vi "test8-AsteriskWildcardStatusRegistration.vi"(8 "error in (no error)":errorcluster, 11 "TestCase in":refnum<class "testcase-CSMBroadcast.lvclass">) -> (0 "error out":errorcluster, 3 "TestCase out":refnum<class "testcase-CSMBroadcast.lvclass">)   [LabVIEW 2017, in "testcase-CSMBroadcast.lvclass"]
uses:
  testcase-CSMBroadcast.lvclass
  0c20cacf-7d77-4f8e-aec5-f22e7d09936d.vi
  26de337d-8090-412f-9da5-e117a55d4726.vi
  de10340a-d592-45ad-b055-7fa7b377c551.vi
  e3eae2f8-d8ce-4adb-8167-9a417250fce1.vi
  a4d00e00-a9ed-4631-bf53-269bf71f16fc.vi
  src/user.lib/_NEVSTOP/Communicable State Machine(CSM)/AdvanceAPI/CSM - Revert Arguments-Safe String.vi
  src/user.lib/_NEVSTOP/Communicable State Machine(CSM)/AdvanceAPI/CSM - Make String Arguments Safe.vi
  src/user.lib/_NEVSTOP/Communicable State Machine(CSM)/AdvanceAPI/CSM - Break Down Multiple States String.vi
  src/user.lib/_NEVSTOP/Communicable State Machine(CSM)/AdvanceAPI/CSM - Compact Multiple States.vi
  src/user.lib/_NEVSTOP/Communicable State Machine(CSM)/AdvanceAPI/CSM - Keywords.vi
  src/user.lib/_NEVSTOP/Communicable State Machine(CSM)/_Shared/Trim Single-line Text.vi
  src/user.lib/_NEVSTOP/Communicable State Machine(CSM)/AdvanceAPI/CSM - Set Module Attribute.vi
  src/user.lib/_NEVSTOP/Communicable State Machine(CSM)/AdvanceAPI/CSM - Get Module Attribute.vi
  <vilib>/addons/_JKI Toolkits/VI Tester/TestCase.llb/TestCase.lvclass
  src/user.lib/_NEVSTOP/Communicable State Machine(CSM)/Communicable State Machine.lvlib
  CSM/CSM-Testcase.lvlib
  C:/Program Files (x86)/National Instruments/LabVIEW 2017/vi.lib/addons/_JKI Toolkits/VI Tester/TestCase.llb/TestCase.lvclass
panel:
  out "Execution Times":i32
  out "State History":string
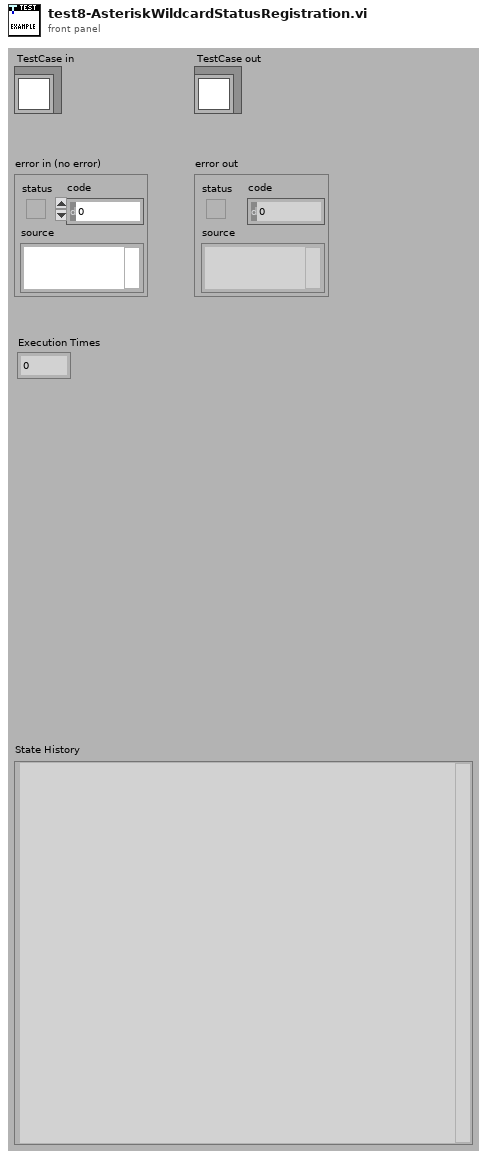
[diagram p1: front panel]
types:
  T1 = enum32{"Invalid", "Standard", "Closed", "Hidden", "Minimized", "Maximized"}
  T2 = enum32{"invalid app kind", "Development System", "Run Time System", "Student Edition", "Embedded LabVIEW", "Evaluation", "Custom"}
  T3 = typedef "Communicable State Machine.lvlib/_CSM_Response Source Message.ctl" = cluster{"‘State":string, "’Arguments":string, "’Error":errorcluster}
  T4 = cluster{"Current VI Reference":refnum<vi>, "Close Panel on Exit?":bool}
  T5 = cluster{"Core":cluster{"Current VI Reference":refnum<vi>, "Close Panel on Exit?":bool}, "Your Boolean data":bool, "Your string data":string, "TestData":i32}
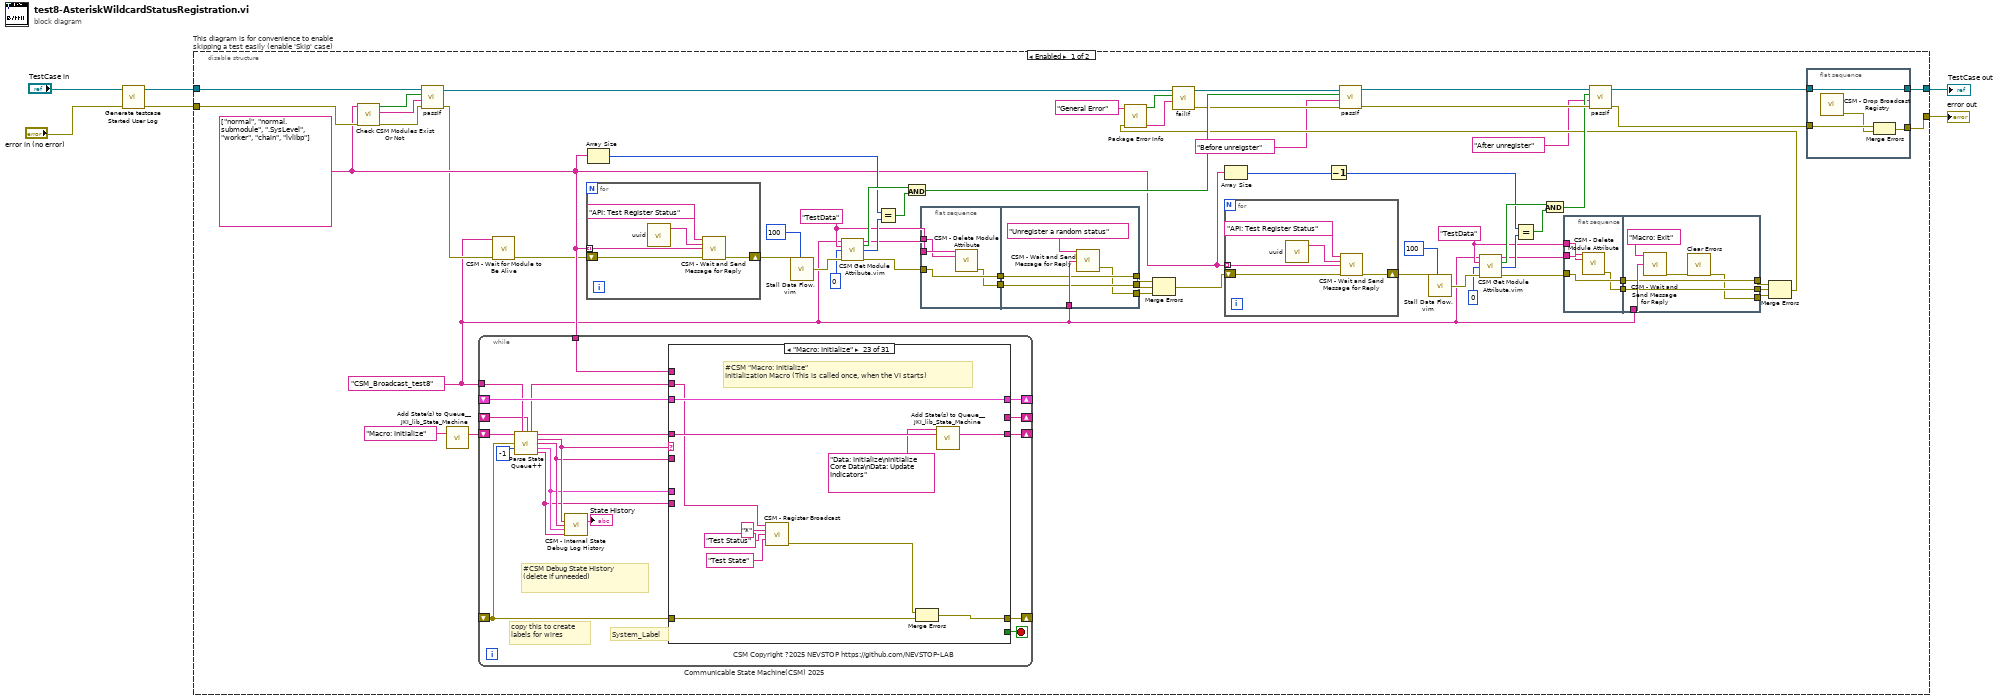
[diagram p0: block diagram]
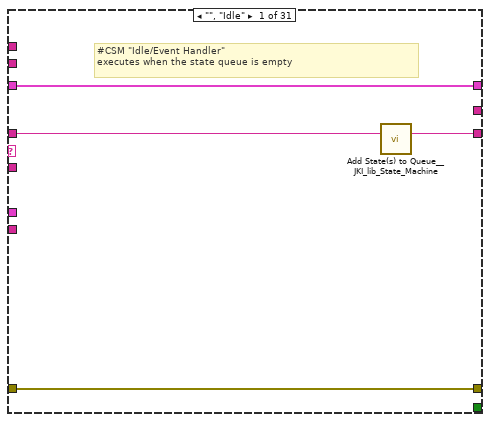
[diagram p2: hidden frame]
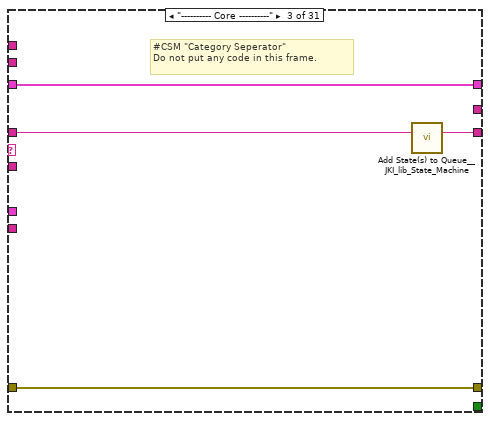
[diagram p4: hidden frame]
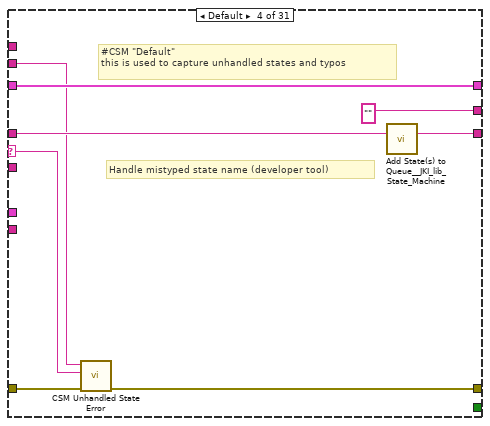
[diagram p5: hidden frame]
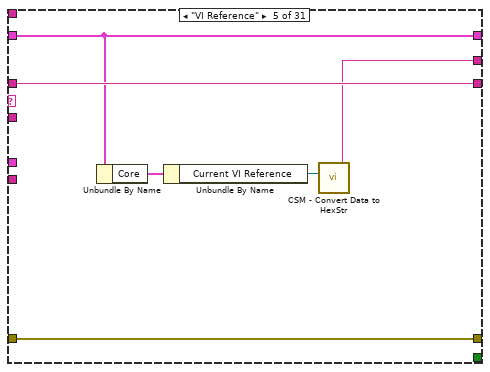
[diagram p6: hidden frame]
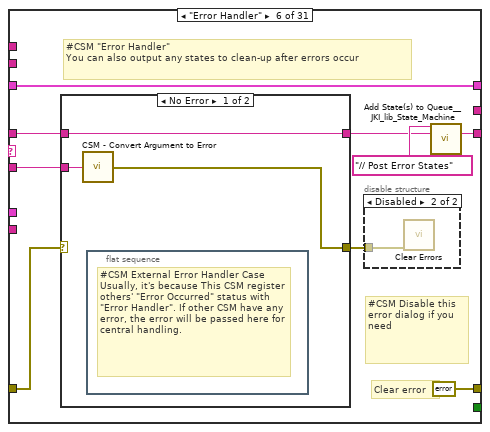
[diagram p7: hidden frame]
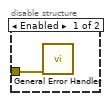
[diagram p8: hidden frame]
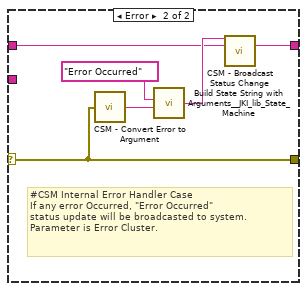
[diagram p9: hidden frame]
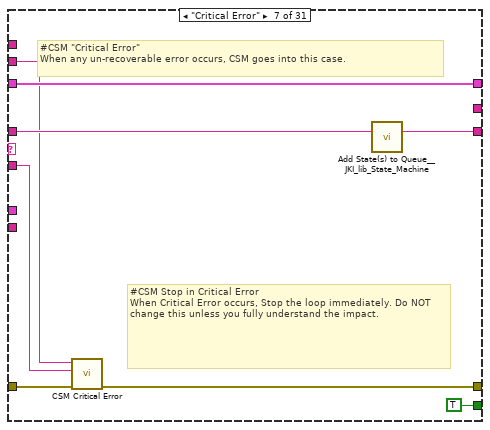
[diagram p10: hidden frame]
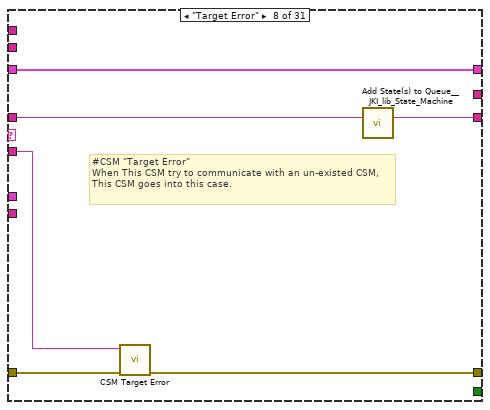
[diagram p11: hidden frame]
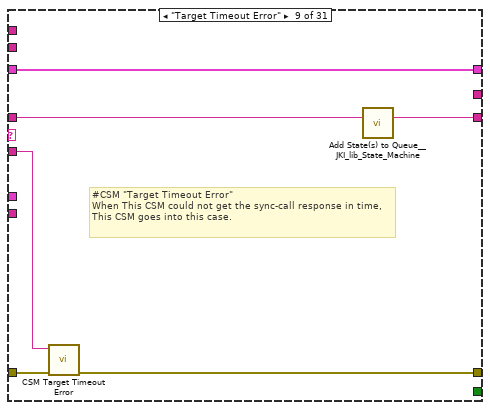
[diagram p12: hidden frame]
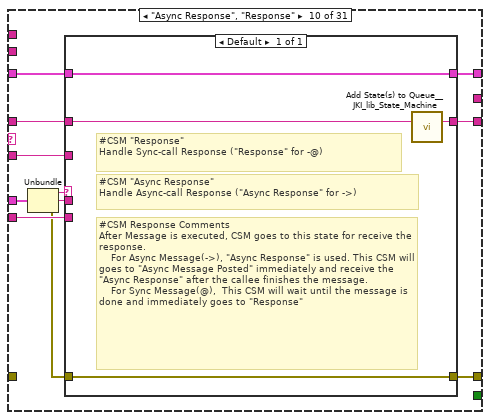
[diagram p13: hidden frame]
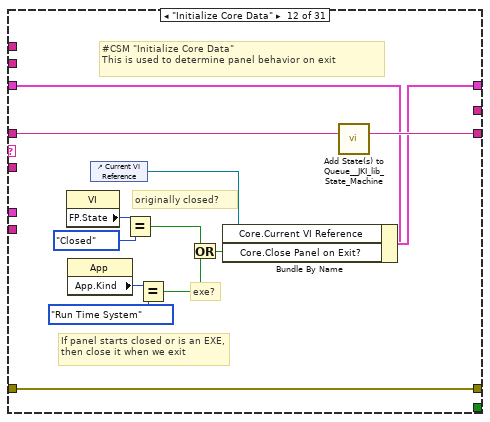
[diagram p15: hidden frame]
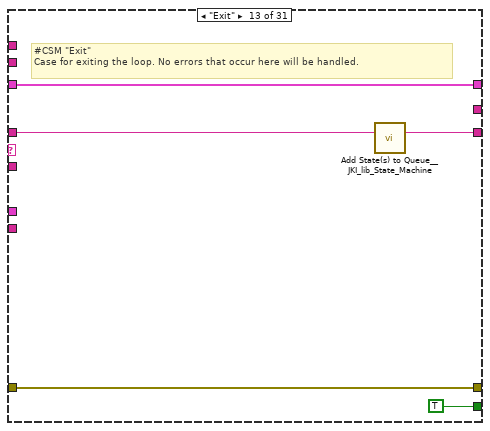
[diagram p16: hidden frame]
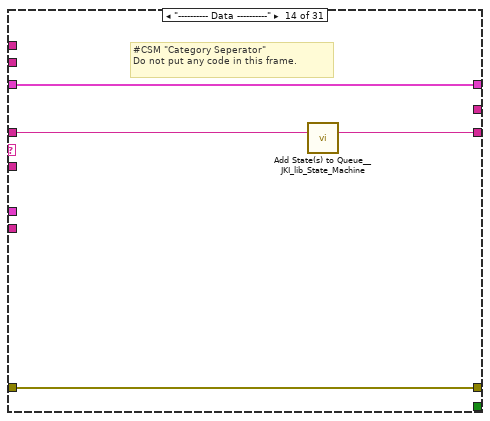
[diagram p17: hidden frame]
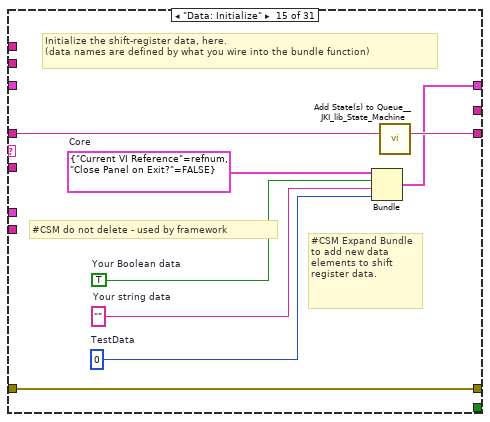
[diagram p18: hidden frame]
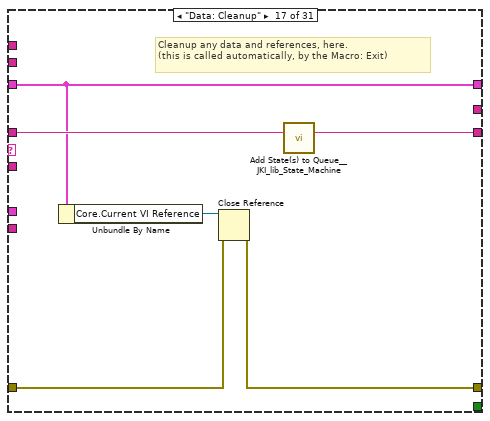
[diagram p20: hidden frame]
diagram:
  n1 = call "Generate testcase Started User Log.vi"("Error In"="error in (no error)") -> ("error out"=w1:errorcluster)  [unwired: 10 in]
  n2 = disable-structure "This diagram is for convenience to enable skipping a test easily (enable 'Skip' case)" shown="Enabled" {
    disable-tunnel: "TestCase in" -> [w24 w420]
    disable-tunnel: [w19 w418] -> w2
    disable-tunnel: [w18 w419] -> w4
    disable-tunnel: w1 -> [w23 w417]
    frame Enabled {
      w33 = "TestData" ("Attribute")
      w55 = "TestData" ("Attribute")
      w6 = "CSM_Broadcast_test8" ("Name (\"\" to Use UUID)")
      w22 = string[] ["normal", "normal.submodule", ".SysLevel", "worker", "chain", "lvlibp"]
      n3 = call "Check CSM Modules Exist Or Not.vi"("error in"=w23, "CSM names in"=w22) -> ("error out"=w25:errorcluster, "Debug string"=w26:string, "All Modules Exist?"=w27:bool)  [unwired: 7 in]
      n4 = call-dynamic "passIf.vi"("error in (no error)"=w25, "message (\"\")"=w26, "pass"=w27, "TestCase in"=w24) -> ("error out"=w8:errorcluster, "TestCase out"=w16:refnum<class "testcase-CSMBroadcast.lvclass">)  [unwired: 6 in]
      n5 = call <vilib>:"Add State(s) to Queue__JKI_lib_State_Machine.vi"("State(s) in (\"\")"="Macro: Initialize" ("Init State(\"Macro: Initialize\")")) -> ("States Out"=w66:string)  [unwired: 14 in]
      n6 = while "Communicable State Machine(CSM) 2025" {
        shift-right: [w109] -> _
        shift-left: _ -> [w108]
        shift-right: [w112] -> _
        shift-left: _ -> [w107]
        shift-right: [w111] -> _
        shift-left: w66 -> [w113]
        tunnel: w6 -> [w105]
        shift-right: [w106] -> _
        shift-left: _ -> [w99]
        tunnel: w22 -> [w96]
        stop <- w110 stop-if-true
        # "#CSM Debug State History\n(delete if unneeded)"
        # "copy this to create labels for wires"
        # "System_Label"
        # "CSM Copyright ?2025 NEVSTOP https://github.com/NEVSTOP-LAB"
        n7 = call "Parse State Queue++.vi"("State Queue"=w113, "Name (\"\" to Use UUID)"=w105, "Response Arguments"=w99, "Previous Error"=w107, "Dequeue (1 ms)"=-1 ("Timeout")) -> ("Name Used"=w100:string, "Remaining States"=w114:string, "Current State"=w104:string, "Arguments"=w103:string, "Additional Information"=w102:T3, "Source CSM"=w101:string)  [unwired: 5 in]
        n8 = call "CSM - Internal State Debug Log History.vi"("State"=w104, "Arguments (\"\")"=w103, ">> Response Source Message >>"=w102, "Source (\"\")"=w101) -> ("Debug Log"=→"State History":string)  [unwired: 11 in]
        n9 = case shown="\"Macro: Initialize\"" w104 {
          selector: w104 -> [_ _ _ w128 _ _ _ _ _ _ _ _ _ _ _ _ _ _ _ _ _ _ _ _ _ _ _ _ _ _ _]
          tunnel: w114 -> [w115 w120 w125 w132 w138 w144 w165 w171 w177 w185 w196 w210 w215 w219 w227 w229 w236 w240 w244 w250 w265 w334 w345 w358 w360 w364 w369 w376 w380 w391 w411]
          tunnel: w103 -> [_ _ _ _ _ w143 w161 w170 w175 w184 _ _ _ _ _ _ _ _ _ w245 w259 _ _ _ _ _ w367 _ _ _ _]
          tunnel: w108 -> [w116 w119 w122 w130 w137 w147 w166 w172 w178 w187 w195 w203 w213 w216 _ w228 w231 w237 w242 w248 w261 w331 w342 w355 w359 w363 w368 w373 w377 w383 w397]
          tunnel: [w117 w121 w123 w126 w139 errorcluster {"status"=FALSE, "code"=0, "source"=""} ("error out") w162 w168 w174 w190 w197 w207 w212 w217 w224 w230 w232 w238 w241 w246 w262 w332 w336 w347 w361 w365 w370 w374 w378 w385 w399] -> w112
          tunnel: w107 -> [w117 w121 w123 w133 w139 w145 w167 w169 w176 _ w197 w207 w212 w217 w224 w230 w233 w238 w241 w247 w263 w332 w343 w356 w361 w365 w370 w374 w378 w389 w409]
          tunnel: [w118 w120 w124 w131 w138 w140 w164 w173 w179 w186 w196 w209 w214 w218 w226 w229 w235 w239 w243 w249 w264 w333 w344 w357 w360 w364 w369 w375 w379 w390 w410] -> w111
          tunnel: [_ _ _ _ _ _ TRUE _ _ _ _ _ TRUE _ _ _ _ _ _ _ _ _ _ _ _ _ _ _ _ _ _] -> w110
          tunnel: [w116 w119 w122 w130 w137 w147 w166 w172 w178 w188 w195 w208 w213 w216 w225 w228 w231 w237 w242 w248 w261 w331 w342 w355 w359 w363 w368 w373 w377 w387 w395] -> w109
          tunnel: w101 -> [_ _ _ _ _ _ _ _ _ w182 _ _ _ _ _ _ _ _ _ _ _ _ _ _ _ _ _ _ _ _ _]
          tunnel: w102 -> [_ _ _ _ _ _ _ _ _ w189 _ _ _ _ _ _ _ _ _ _ _ _ _ _ _ _ _ _ _ _ _]
          tunnel: [_ _ _ "" w134 _ _ _ _ _ _ _ _ _ _ _ _ _ _ _ _ _ _ _ _ "API1 Response" w366 _ _ _ _] -> w106
          tunnel: w100 -> [_ _ _ w127 _ _ w160 _ _ _ _ _ _ _ _ _ _ _ _ _ _ _ w337 w349 _ _ _ _ _ w386 w406]
          tunnel: w96 -> [_ _ _ _ _ _ _ _ _ _ _ _ _ _ _ _ _ _ _ _ _ _ _ _ _ _ _ _ _ _ w402]
          frame "", "Idle" {
            # "#CSM \"Idle/Event Handler\"\nexecutes when the state queue is empty"
            n10 = call <vilib>:"Add State(s) to Queue__JKI_lib_State_Machine.vi"("State(s) in (\"\")"=w115) -> ("States Out"=w118:string)  [unwired: 14 in]
          }
          frame "CSM Documentation" {
            # "#CSM README FIRST\n\nCommunicable State Machine(CSM) is a LabVIEW application framework that builds upon JKI State Machine(JKISM). It follows the pattern of JKISM and extends the keywords to describe message communication between modules, including concepts such as Sync-Message, Async-Message, Subscription/Unsubscription of status - essential elements for creating reusable code modules. For more information, please visit the CSM wiki: https://nevstop-lab.github.io/CSM-Wiki/\n\nFor instructions on JKI State Machine, visit: http://jki.net/state-machine/\nFor information about CSM, visit: https://github.com/NEVSTOP-LAB"
            # "#CSM \"Documentation\"\nCase for holding CSM Documenation"
          }
          frame "---------- Core ----------" {
            # "#CSM \"Category Seperator\"\nDo not put any code in this frame."
            n11 = call <vilib>:"Add State(s) to Queue__JKI_lib_State_Machine.vi"("State(s) in (\"\")"=w125) -> ("States Out"=w124:string)  [unwired: 14 in]
          }
          frame Default {
            # "#CSM \"Default\"\nthis is used to capture unhandled states and typos"
            # "Handle mistyped state name (developer tool)"
            n12 = call "CSM Unhandled State Error.vi"("error in (no error)"=w133, "Undefined State"=w128, "CSM Name"=w127) -> ("error out"=w126:errorcluster)  [unwired: 8 in]
            n13 = call <vilib>:"Add State(s) to Queue__JKI_lib_State_Machine.vi"("State(s) in (\"\")"=w132) -> ("States Out"=w131:string)  [unwired: 14 in]
          }
          frame "VI Reference" {
            n14 = Unbundle By Name(w137) -> ("Core"=w136:T4)
            n15 = Unbundle By Name(w136) -> ("Current VI Reference"=w135:refnum<vi>)
            n16 = call "CSM - Convert Data to HexStr.vi"("Variant"=w135) -> ("HEX String (0-9,A-F)"=w134:string)  [unwired: 8 in]
          }
          frame "Error Handler" {
            # "#CSM Disable this error dialog if you need"
            # "#CSM \"Error Handler\"\nYou can also output any states to clean-up after errors occur"
            # "Clear error"
            n17 = case shown="No Error" w145 {
              selector: w145 -> [_ w154]
              tunnel: [w153 w156] -> w141
              tunnel: w144 -> [w153 w155]
              tunnel: w143 -> [w152 _]
              tunnel: [w151 w154] -> w146
              frame No Error {
                n18 = call "CSM - Convert Argument to Error.vi"("Argument"=w152) -> ("Error"=w151:errorcluster)  [unwired: 4 in]
                n19 = flat-sequence {
                  frame #0 {
                    # "#CSM External Error Handler Case\nUsually, it's because This CSM register others' \"Error Occurred\" status with \"Error Handler\". If other CSM have any error, the error will be passed here for central handling."
                  }
                }
              }
              frame Error {
                # "#CSM Internal Error Handler Case \nIf any error Occurred, \"Error Occurred\" \nstatus update will be broadcasted to system.\nParameter is Error Cluster."
                n20 = call "CSM - Convert Error to Argument.vi"("Error"=w154) -> ("Argument"=w158:string)  [unwired: 4 in]
                n21 = call <vilib>:"Build State String with Arguments__JKI_lib_State_Machine.vi"("Arguments (\"\")"=w158, "State"="Error Occurred" ("Status with Arguments")) -> ("State with Arguments"=w157:string)  [unwired: 4 in]
                n22 = call "CSM - Broadcast Status Change.vi"("Status With Arguments"=w157, "State Queue"=w155) -> ("Remaining States"=w156:string)  [unwired: 13 in]
              }
            }
            n23 = disable-structure shown="Disabled" {
              disable-tunnel: w146 -> [w149 w150]
              frame Enabled {
                n24 = call <vilib>:"General Error Handler.vi"("error in (no error)"=w149) -> ()  [unwired: 10 in, 5 out]
              }
              frame Disabled {
                n25 = call <vilib>:"Clear Errors.vi"("error in (no error)"=w150) -> ()  [unwired: 5 in, 2 out]
              }
            }
            n26 = call <vilib>:"Add State(s) to Queue__JKI_lib_State_Machine.vi"("State(s) in Front (\"\")"="// Post Error States", "State(s) in (\"\")"=w141) -> ("States Out"=w140:string)  [unwired: 13 in]
          }
          frame "Critical Error" {
            # "#CSM Stop in Critical Error\nWhen Critical Error occurs, Stop the loop immediately. Do NOT change this unless you fully understand the impact."
            # "#CSM \"Critical Error\"\nWhen any un-recoverable error occurs, CSM goes into this case."
            n27 = call "CSM Critical Error.vi"("error in (no error)"=w167, "Arugments (As Reason)"=w161, "CSM Name"=w160) -> ("error out"=w162:errorcluster)  [unwired: 8 in]
            n28 = call <vilib>:"Add State(s) to Queue__JKI_lib_State_Machine.vi"("State(s) in (\"\")"=w165) -> ("States Out"=w164:string)  [unwired: 14 in]
          }
          frame "Target Error" {
            # "#CSM \"Target Error\"\nWhen This CSM try to communicate with an un-existed CSM, This CSM goes into this case."
            n29 = call "CSM Target Error.vi"("error in (no error)"=w169, "Arguments (As CSM Name)"=w170) -> ("error out"=w168:errorcluster)  [unwired: 9 in]
            n30 = call <vilib>:"Add State(s) to Queue__JKI_lib_State_Machine.vi"("State(s) in (\"\")"=w171) -> ("States Out"=w173:string)  [unwired: 14 in]
          }
          frame "Target Timeout Error" {
            # "#CSM \"Target Timeout Error\"\nWhen This CSM could not get the sync-call response in time, This CSM goes into this case."
            n31 = call "CSM Target Timeout Error.vi"("error in (no error)"=w176, "Arguments (As CSM Name)"=w175) -> ("error out"=w174:errorcluster)  [unwired: 9 in]
            n32 = call <vilib>:"Add State(s) to Queue__JKI_lib_State_Machine.vi"("State(s) in (\"\")"=w177) -> ("States Out"=w179:string)  [unwired: 14 in]
          }
          frame "Async Response", "Response" {
            n33 = Unbundle(w189) -> ("‘State"=w183:string, "’Arguments"=w181:string, "’Error"=w180:errorcluster)
            n34 = case shown="Default" w183 {
              tunnel: [w194] -> w190
              tunnel: w180 -> [w194]
              tunnel: [w193] -> w188
              tunnel: w187 -> [w193]
              tunnel: [w191] -> w186
              tunnel: w185 -> [w192]
              tunnel: w184 -> [_]
              tunnel: w182 -> [_]
              tunnel: w181 -> [_]
              frame Default {
                # "#CSM Response Comments\nAfter Message is executed, CSM goes to this state for receive the response.\n    For Async Message(->), \"Async Response\" is used. This CSM will goes to \"Async Message Posted\" immediately and receive the \"Async Response\" after the callee finishes the message.\n    For Sync Message(@),  This CSM will wait until the message is done and immediately goes to \"Response\""
                # "#CSM \"Async Response\"\nHandle Async-call Response (\"Async Response\" for ->)"
                # "#CSM \"Response\"\nHandle Sync-call Response (\"Response\" for -@)"
                n35 = call <vilib>:"Add State(s) to Queue__JKI_lib_State_Machine.vi"("State(s) in (\"\")"=w192) -> ("States Out"=w191:string)  [unwired: 14 in]
              }
            }
          }
          frame "Async Message Posted" {
            # "#CSM \"Async Message Posted\"\nAfter Async Message is posted (-> or ->| ), CSM goes to this state for post-action.\nYou can use Argument - State to tell which Async Message is called."
          }
          frame "Initialize Core Data" {
            # "#CSM \"Initialize Core Data\"\nThis is used to determine panel behavior on exit"
            # "originally closed?"
            # "exe?"
            # "If panel starts closed or is an EXE, then close it when we exit"
            n36 = property class="VI"() -> ("FP.State"=w200:T1)  [unwired: 2 in, 2 out]
            n37 = property class="App"() -> ("App.Kind"=w206:T2)  [unwired: 2 in, 2 out]
            n38 = control-ref of="Current VI Reference"() -> (w201:refnum<vi>)
            n39 = Equal?(x=w200, y=T1."Closed" ("Front Panel Window:State")) -> (x = y?=w198:bool)
            n40 = Equal?(x=w206, y=T2."Run Time System" ("Application:Kind")) -> (x = y?=w204:bool)
            n41 = Or(x=w198, y=w204) -> (x .or. y?=w202:bool)
            n42 = Bundle By Name(cluster=w203, "Core.Current VI Reference"=w201, "Core.Close Panel on Exit?"=w202) -> (w208:T5)
            n43 = call <vilib>:"Add State(s) to Queue__JKI_lib_State_Machine.vi"("State(s) in (\"\")"=w210) -> ("States Out"=w209:string)  [unwired: 14 in]
          }
          frame "Exit" {
            # "#CSM \"Exit\"\nCase for exiting the loop. No errors that occur here will be handled."
            n44 = call <vilib>:"Add State(s) to Queue__JKI_lib_State_Machine.vi"("State(s) in (\"\")"=w215) -> ("States Out"=w214:string)  [unwired: 14 in]
          }
          frame "---------- Data ----------" {
            # "#CSM \"Category Seperator\"\nDo not put any code in this frame."
            n45 = call <vilib>:"Add State(s) to Queue__JKI_lib_State_Machine.vi"("State(s) in (\"\")"=w219) -> ("States Out"=w218:string)  [unwired: 14 in]
          }
          frame "Data: Initialize" {
            w220 = 0  # TestData
            w221 = T4 {"Current VI Reference"=refnum, "Close Panel on Exit?"=FALSE}  # Core
            w223 = TRUE  # Your Boolean data
            w222 = ""  # Your string data
            # "#CSM do not delete - used by framework"
            # "#CSM Expand Bundle to add new data elements to shift register data."
            # "Initialize the shift-register data, here.\n(data names are defined by what you wire into the bundle function)"
            n46 = Bundle("Core"=w221, "Your Boolean data"=w223, "Your string data"=w222, "TestData"=w220) -> (w225:T5)  [unwired: 1 in]
            n47 = call <vilib>:"Add State(s) to Queue__JKI_lib_State_Machine.vi"("State(s) in (\"\")"=w227) -> ("States Out"=w226:string)  [unwired: 14 in]
          }
          frame "Data: Update Indicators" {
          }
          frame "Data: Cleanup" {
            # "Cleanup any data and references, here.\n(this is called automatically, by the Macro: Exit)"
            n48 = Unbundle By Name(w231) -> ("Core.Current VI Reference"=w234:refnum<vi>)
            n49 = Close Reference(reference=w234, error in (no error)=w233) -> (error out=w232:errorcluster)
            n50 = call <vilib>:"Add State(s) to Queue__JKI_lib_State_Machine.vi"("State(s) in (\"\")"=w236) -> ("States Out"=w235:string)  [unwired: 14 in]
          }
          frame "---------- UI ----------" {
            # "#CSM \"Category Seperator\"\nDo not put any code in this frame."
            n51 = call <vilib>:"Add State(s) to Queue__JKI_lib_State_Machine.vi"("State(s) in (\"\")"=w240) -> ("States Out"=w239:string)  [unwired: 14 in]
          }
          frame "UI: Initialize" {
            # "#CSM \"UI: Initialize\"\nInitialize the User Interface, here.\n(this is called automatically, by the Macro: Init)"
            n52 = call <vilib>:"Add State(s) to Queue__JKI_lib_State_Machine.vi"("State(s) in (\"\")"=w244) -> ("States Out"=w243:string)  [unwired: 14 in]
          }
          frame "UI: Cursor Set" {
            # "#CSM \"UI: Cursor Set\"\nSet and Unset Cursor Busy.\n(Usage: \"UI: Cursor Set >> Busy|Idle\")"
            # "Argument"
            n53 = disable-structure shown="TARGET_TYPE!=Windows" {
              disable-tunnel: w247 -> [w253 w258]
              disable-tunnel: [w252 w258] -> w246
              disable-tunnel: w245 -> [w251 _]
              frame condition #0 (active) {
                n54 = case shown="\"Idle\", Default" w251 {
                  tunnel: w253 -> [w255 w257]
                  tunnel: [w254 w256] -> w252
                  frame "Idle", Default {
                    n55 = call <vilib>:"Unset Busy.vi"("error in (no error)"=w255) -> ("error out"=w254:errorcluster)  [unwired: 10 in]
                  }
                  frame "Busy" {
                    n56 = call <vilib>:"Set Busy.vi"("error in (no error)"=w257) -> ("error out"=w256:errorcluster)  [unwired: 9 in, 1 out]
                  }
                }
              }
              frame condition #1 {
              }
            }
            n57 = call <vilib>:"Add State(s) to Queue__JKI_lib_State_Machine.vi"("State(s) in (\"\")"=w250) -> ("States Out"=w249:string)  [unwired: 14 in]
          }
          frame "UI: Front Panel State" {
            # "#CSM \"UI: Front Panel State\"\nSet Front Panel Open or Closed\n(Usage: \"UI: Front Panel State >> Open|Close\")"
            # "Argument"
            n58 = Unbundle By Name(w261) -> ("Core.Current VI Reference"=w260:refnum<vi>)
            n59 = call <vilib>:"Add State(s) to Queue__JKI_lib_State_Machine.vi"("State(s) in (\"\")"=w265) -> ("States Out"=w264:string)  [unwired: 14 in]
            n60 = case shown="\"Close\", \"Closed\"" w259 {
              tunnel: w263 -> [w271 w286 w297 w310 w323]
              tunnel: [w273 w287 w299 w312 w325] -> w262
              tunnel: w260 -> [w272 w284 w298 w311 w324]
              frame "Open", "Standard", Default {
                w266 = T1."Standard" ("State")
                n61 = property class="VI"(reference=w272, error in=w271) -> (reference out=w269:refnum<vi>, error out=w270:errorcluster, "FP.State"=w268:T1)
                n62 = Not Equal?(x=w268, y=w266) -> (x != y?=w267:bool)
                n63 = case shown="True" w267 {
                  tunnel: [w277 w279] -> w273
                  tunnel: w270 -> [w276 w279]
                  tunnel: w269 -> [w275 _]
                  tunnel: w266 -> [w274 _]
                  frame True {
                    n64 = invoke class="VI" method="FP.Open"(reference=w275, error in=w276, "Activate"=TRUE, "State"=w274) -> (error out=w277:errorcluster)  [unwired: 1 in, 4 out]
                  }
                  frame False {
                  }
                }
              }
              frame "Close", "Closed" {
                n65 = property class="VI"(reference=w284, error in=w286) -> (reference out=w283:refnum<vi>, error out=w285:errorcluster, "FP.State"=w281:T1)
                n66 = Not Equal?(x=w281, y=T1."Closed" ("Front Panel Window:State")) -> (x != y?=w280:bool)
                n67 = case shown="False" w280 {
                  tunnel: [w288 w291] -> w287
                  tunnel: w285 -> [w288 w290]
                  tunnel: w283 -> [_ w289]
                  frame False {
                  }
                  frame True {
                    n68 = invoke class="VI" method="FP.Close"(reference=w289, error in=w290) -> (error out=w291:errorcluster)  [unwired: 1 in, 2 out]
                  }
                }
              }
              frame "Hidden", "Hide" {
                w292 = T1."Hidden" ("State")
                n69 = property class="VI"(reference=w298, error in=w297) -> (reference out=w295:refnum<vi>, error out=w296:errorcluster, "FP.State"=w294:T1)
                n70 = Not Equal?(x=w294, y=w292) -> (x != y?=w293:bool)
                n71 = case shown="True" w293 {
                  tunnel: [w303 w304] -> w299
                  tunnel: w296 -> [w302 w304]
                  tunnel: w295 -> [w301 _]
                  tunnel: w292 -> [w300 _]
                  frame True {
                    n72 = invoke class="VI" method="FP.Open"(reference=w301, error in=w302, "State"=w300) -> (error out=w303:errorcluster)  [unwired: 2 in, 4 out]
                  }
                  frame False {
                  }
                }
              }
              frame "Minimize", "Minimized" {
                w305 = T1."Minimized" ("State")
                n73 = property class="VI"(reference=w311, error in=w310) -> (reference out=w308:refnum<vi>, error out=w309:errorcluster, "FP.State"=w307:T1)
                n74 = Not Equal?(x=w307, y=w305) -> (x != y?=w306:bool)
                n75 = case shown="True" w306 {
                  tunnel: [w316 w317] -> w312
                  tunnel: w309 -> [w315 w317]
                  tunnel: w308 -> [w314 _]
                  tunnel: w305 -> [w313 _]
                  frame True {
                    n76 = invoke class="VI" method="FP.Open"(reference=w314, error in=w315, "State"=w313) -> (error out=w316:errorcluster)  [unwired: 2 in, 4 out]
                  }
                  frame False {
                  }
                }
              }
              frame "Maximize", "Maximized" {
                w318 = T1."Maximized" ("State")
                n77 = property class="VI"(reference=w324, error in=w323) -> (reference out=w321:refnum<vi>, error out=w322:errorcluster, "FP.State"=w320:T1)
                n78 = Not Equal?(x=w320, y=w318) -> (x != y?=w319:bool)
                n79 = case shown="True" w319 {
                  tunnel: [w329 w330] -> w325
                  tunnel: w322 -> [w328 w330]
                  tunnel: w321 -> [w327 _]
                  tunnel: w318 -> [w326 _]
                  frame True {
                    n80 = invoke class="VI" method="FP.Open"(reference=w327, error in=w328, "State"=w326) -> (error out=w329:errorcluster)  [unwired: 2 in, 4 out]
                  }
                  frame False {
                  }
                }
              }
            }
          }
          frame "---------- Macro ----------" {
            # "#CSM \"Category Seperator\"\nDo not put any code in this frame."
            n81 = call <vilib>:"Add State(s) to Queue__JKI_lib_State_Machine.vi"("State(s) in (\"\")"=w334) -> ("States Out"=w333:string)  [unwired: 14 in]
          }
          frame "Macro: Initialize" {
            # "#CSM \"Macro: Initialize\"\nInitialization Macro (This is called once, when the VI starts)"
            n82 = call "CSM - Register Broadcast.vi"("CSM Name(Empty for Broadcast Event)"=w337, "Source CSM Name (* as Default)"="*", "Trigger"="Test Status" ("Status"), "API (If \"\", Same as Trigger)"="Test State" ("Response Message (If \"\", Same as Source Message)")) -> ("error out"=w335:errorcluster)  [unwired: 10 in, 1 out]
            n83 = Merge Errors(w335, w343) -> (w336:errorcluster)
            n84 = call <vilib>:"Add State(s) to Queue__JKI_lib_State_Machine.vi"("State(s) in Front (\"\")"="Data: Initialize\nInitialize Core Data\nData: Update Indicators", "State(s) in (\"\")"=w345) -> ("States Out"=w344:string)  [unwired: 13 in]
          }
          frame "Macro: Exit" {
            # "#CSM \"Macro: Exit\"\nExit Macro (This is called once, when the VI exits)"
            n85 = call "CSM - Unregister Broadcast.vi"("CSM Name(Empty for Broadcast Event)"=w349, "Source CSM Name (* as Default)"="*", "Trigger"="Test Status" ("Status"), "API (\"*\" as Default)"="Test State" ("Response Message (If \"\", Same as Source Message)")) -> ("error out"=w346:errorcluster)  [unwired: 10 in, 1 out]
            n86 = call <vilib>:"Add State(s) to Queue__JKI_lib_State_Machine.vi"("State(s) in Front (\"\")"="//Exit Sub-Modules ", "State(s) at Back (\"\")"="Data: Cleanup\nExit") -> ("States Out"=w353:string)  [unwired: 13 in]
            n87 = Merge Errors(w346, w356) -> (w347:errorcluster)
            n88 = call <vilib>:"Add State(s) to Queue__JKI_lib_State_Machine.vi"("State(s) in Front (\"\")"=w353, "State(s) in (\"\")"=w358) -> ("States Out"=w357:string)  [unwired: 13 in]
          }
          frame "---------- API ----------" {
            # "#CSM \"Category Seperator\"\nDo not put any code in this frame."
          }
          frame "API: API1" {
            # "#CSM API Example\nCopy/Rename this case for your own API"
            # "#CSM Response\nConnect this to return the response of your API"
            # "#CSM >> Msg/Rep's CSM >>\nIf you need to tell who triggered this state , use this string. If it's this case itself, this string is \"\"."
            # "#CSM >> Arguments >>\nDeal with the parameter if any"
          }
          frame "API: API2" {
            # "#CSM API Example\nCopy/Rename this case for your own API"
            # "unpack Hex String  to Variant\nif complex parameter is needed."
            n89 = call "CSM - Convert HexStr to Data.vi"("HEX String"=w367) -> ()  [unwired: 7 in, 2 out]
            n90 = disable-structure shown="Disabled" {
              disable-tunnel: [w371 "API2 Response"] -> w366
              frame Disabled {
                # "pack variant to hexstr \nif complex response is needed."
                # "complex Response"
                n91 = call "CSM - Convert Data to HexStr.vi"() -> ("HEX String (0-9,A-F)"=w371:string)  [unwired: 9 in]
              }
              frame Enabled {
              }
            }
          }
          frame "---------- Action ----------" {
            # "#CSM \"Category Seperator\"\nDo not put any code in this frame."
            n92 = call <vilib>:"Add State(s) to Queue__JKI_lib_State_Machine.vi"("State(s) in (\"\")"=w376) -> ("States Out"=w375:string)  [unwired: 14 in]
          }
          frame "Action: action1" {
            # "#CSM \"Internal State\"\nThis category is used for holding internal states"
            n93 = call <vilib>:"Add State(s) to Queue__JKI_lib_State_Machine.vi"("State(s) in (\"\")"=w380) -> ("States Out"=w379:string)  [unwired: 14 in]
          }
          frame "Test State" {
            n94 = Unbundle By Name(w383) -> ("TestData"=w388:i32)
            n95 = disable-structure shown="Enabled" {
              frame Disabled {
                n96 = feedback #1(0 ("y")) -> (w393:i32)
                n97 = Increment(x=w393) -> (x+1=w392:i32)
                "Execution Times" <- w392
                n98 = feedback-in #1(w392) -> ()
              }
              frame Enabled {
              }
            }
            n99 = Increment(x=w388) -> (x+1=w381:i32)
            n100 = Bundle By Name(cluster=w383, "TestData"=w381) -> (w387:T5)
            n101 = call "CSM Set Module Attribute.vim"("CSM Name"=w386, "Attribute"="TestData", "Value"=w381) -> ("error out"=w384:errorcluster)  [unwired: 9 in, 3 out]
            n102 = call <vilib>:"Add State(s) to Queue__JKI_lib_State_Machine.vi"("State(s) in (\"\")"=w391) -> ("States Out"=w390:string)  [unwired: 14 in]
            n103 = Merge Errors(w389, w384) -> (w385:errorcluster)
          }
          frame "Unregister a random status" {
            n104 = Random Number (0-1)() -> (number: 0 to 1=w404:dbl)
            n105 = Array Size(array=w402) -> (size(s)=w405:i32)
            n106 = Multiply(x=w405, y=w404) -> (x*y=w403:dbl)
            n107 = Bundle By Name(cluster=w397, "TestData"=0) -> (w395:T5)
            n108 = Round Toward -Infinity(1:w403) -> (0:w401:dbl)
            n109 = Index Array(array=w402, index=w401) -> (element=w400:string)
            n110 = call "CSM - Unregister Broadcast.vi"("CSM Name(Empty for Broadcast Event)"=w406, "Source CSM Name (* as Default)"=w400, "Trigger"="Test Status" ("Status"), "API (\"*\" as Default)"="Test State" ("Response Message (If \"\", Same as Source Message)")) -> ("error out"=w398:errorcluster)  [unwired: 10 in, 1 out]
            n111 = Merge Errors(w409, w398) -> (w399:errorcluster)
            n112 = call <vilib>:"Add State(s) to Queue__JKI_lib_State_Machine.vi"("State(s) in (\"\")"=w411) -> ("States Out"=w410:string)  [unwired: 14 in]
          }
        }
      }
      n113 = call "CSM - Wait for Module to Be Alive.vi"("CSM Name"=w6, "error in (no error)"=w8) -> ("error out"=w7:errorcluster)  [unwired: 11 in, 2 out]
      n114 = for {
        tunnel: w22 -> [w414] mode=indexing
        shift-right: [w413] -> w64
        shift-left: w7 -> [w412]
        n115 = call "uuid.vi"() -> ("UUID"=w415:string)  [unwired: 11 in]
        n116 = call "CSM - Wait and Send Message for Reply.vi"("State"="API: Test Register Status", "Arguments (\"\")"=w415, "Target Module"=w414, "Error In (No Error)"=w412) -> ("error out"=w413:errorcluster)  [unwired: 8 in, 3 out]
      }
      n117 = Array Size(array=w22) -> (size(s)=w59:i32)
      n118 = call "Stall Data Flow.vim"("value in"=w64, "milliseconds to wait"=u32 100) -> ("value out"=w63:errorcluster)  [unwired: 1 out]
      n119 = call "CSM Get Module Attribute.vim"("CSM Name"=w6, "Attribute"=w55, "Default Value (Empty Variant)"=0 ("x+1"), "Error In"=w63) -> ("CSM Name (Dup)"=w56:string, "Found"=w61:bool, "Value"=w60:i32, "error out"=w54:errorcluster)  [unwired: 7 in, 1 out]
      n120 = Equal?(x=w59, y=w60) -> (x = y?=w58:bool)
      n121 = And(x=w61, y=w58) -> (x .and. y?=w57:bool)
      n122 = flat-sequence {
        tunnel: w56 -> [w90]
        tunnel: w55 -> [w89]
        tunnel: w54 -> [w88]
        tunnel: [w88] -> w53
        tunnel: [w87] -> w52
        tunnel: w6 -> [w94]
        tunnel: w53 -> [w93]
        tunnel: w52 -> [w92]
        tunnel: [w93] -> w51
        tunnel: [w92] -> w50
        tunnel: [w91] -> w49
        frame #0 {
          n123 = call "CSM - Delete Module Attribute.vi"("CSM Name"=w90, "Attribute"=w89) -> ("error out"=w87:errorcluster)  [unwired: 10 in, 3 out]
        }
        frame #1 {
          n124 = call "CSM - Wait and Send Message for Reply.vi"("State"="Unregister a random status", "Target Module"=w94) -> ("error out"=w91:errorcluster)  [unwired: 10 in, 3 out]
        }
      }
      n125 = Merge Errors(w51, w50, w49) -> (w41:errorcluster)
      n126 = for {
        tunnel: w22 -> [w84] mode=indexing
        shift-right: [w83] -> w47
        shift-left: w41 -> [w82]
        n127 = call "uuid.vi"() -> ("UUID"=w85:string)  [unwired: 11 in]
        n128 = call "CSM - Wait and Send Message for Reply.vi"("State"="API: Test Register Status", "Arguments (\"\")"=w85, "Target Module"=w84, "Error In (No Error)"=w82) -> ("error out"=w83:errorcluster)  [unwired: 8 in, 3 out]
      }
      n129 = Array Size(array=w22) -> (size(s)=w40:i32)
      n130 = Decrement(x=w40) -> (x-1=w39:i32)
      n131 = call "Stall Data Flow.vim"("value in"=w47, "milliseconds to wait"=u32 100) -> ("value out"=w46:errorcluster)  [unwired: 1 out]
      n132 = call "CSM Get Module Attribute.vim"("CSM Name"=w6, "Attribute"=w33, "Default Value (Empty Variant)"=0 ("x+1"), "Error In"=w46) -> ("CSM Name (Dup)"=w34:string, "Found"=w44:bool, "Value"=w43:i32, "error out"=w32:errorcluster)  [unwired: 7 in, 1 out]
      n133 = Equal?(x=w39, y=w43) -> (x = y?=w42:bool)
      n134 = And(x=w44, y=w42) -> (x .and. y?=w28:bool)
      n135 = flat-sequence {
        tunnel: w34 -> [w75]
        tunnel: w33 -> [w74]
        tunnel: w32 -> [w73]
        tunnel: [w73] -> w36
        tunnel: [w72] -> w35
        tunnel: w6 -> [w80]
        tunnel: w36 -> [w79]
        tunnel: w35 -> [w78]
        tunnel: [w79] -> w31
        tunnel: [w78] -> w30
        tunnel: [w76] -> w29
        frame #0 {
          n136 = call "CSM - Delete Module Attribute.vi"("CSM Name"=w75, "Attribute"=w74) -> ("error out"=w72:errorcluster)  [unwired: 10 in, 3 out]
        }
        frame #1 {
          n137 = call "CSM - Wait and Send Message for Reply.vi"("State"="Macro: Exit", "Target Module"=w80) -> ("error out"=w77:errorcluster)  [unwired: 10 in, 3 out]
          n138 = call <vilib>:"Clear Errors.vi"("error in (no error)"=w77) -> ("error out"=w76:errorcluster)  [unwired: 5 in, 1 out]
        }
      }
      n139 = Merge Errors(w31, w30, w29) -> (w12:errorcluster)
      n140 = call "Package Error Info.vi"("error in"=w12, "String in"="General Error") -> ("packed error info out"=w13:string, "error status"=w17:bool)  [unwired: 8 in]
      n141 = call-dynamic "failIf.vi"("message (\"\")"=w13, "fail"=w17, "TestCase in"=w16) -> ("error out"=w14:errorcluster, "TestCase out"=w15:refnum<class "testcase-CSMBroadcast.lvclass">)  [unwired: 7 in]
      n142 = call-dynamic "passIf.vi"("error in (no error)"=w14, "message (\"\")"="Before unreigster" ("message (\"\")"), "pass"=w57, "TestCase in"=w15) -> ("error out"=w38:errorcluster, "TestCase out"=w37:refnum<class "testcase-CSMBroadcast.lvclass">)  [unwired: 6 in]
      n143 = call-dynamic "passIf.vi"("error in (no error)"=w38, "message (\"\")"="After unregister" ("message (\"\")"), "pass"=w28, "TestCase in"=w37) -> ("error out"=w20:errorcluster, "TestCase out"=w21:refnum<class "testcase-CSMBroadcast.lvclass">)  [unwired: 6 in]
      n144 = flat-sequence {
        tunnel: w20 -> [w71]
        tunnel: [w70] -> w18
        tunnel: w21 -> [w68]
        tunnel: [w68] -> w19
        frame #0 {
          n145 = call "CSM - Drop Broadcast Registry.vi"() -> ("error out"=w69:errorcluster)  [unwired: 15 in]
          n146 = Merge Errors(w71, w69) -> (w70:errorcluster)
        }
      }
    }
    frame Disabled {
      # "skip test result while test is under development"
      n147 = call <vilib>:"skip.vi"("error in (no error)"=w417, "TestCase in"=w420) -> ("error out"=w419:errorcluster, "TestCase out"=w418:refnum<class "testcase-CSMBroadcast.lvclass">)  [unwired: 8 in]
    }
  }
  "error out" <- w4
  "TestCase out" <- w2
